vi "Single Measure Reference Query.vi"(8 "error in":errorcluster, 11 "Instrument Handle In":i32) -> (0 "error out":errorcluster, 1 "Low Reference":dbl, 2 "Mid Reference":dbl, 3 "Instrument Handle Out":i32, 5 "High Reference":dbl)   [LabVIEW 8.6, in "ZTScopeM.lvlib"]
doc: "Query the voltage threshold levels for measurements.\nValues may be in either volts or percent depending on the reference method."
uses:
  ZTScopeM.lvlib
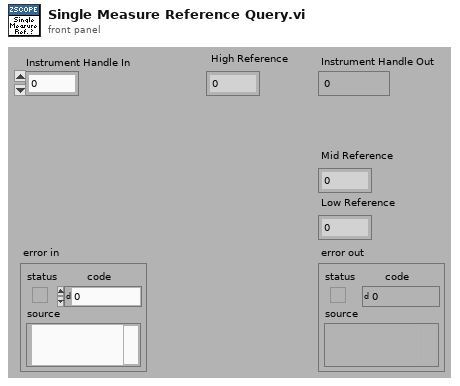
[diagram p1: front panel]
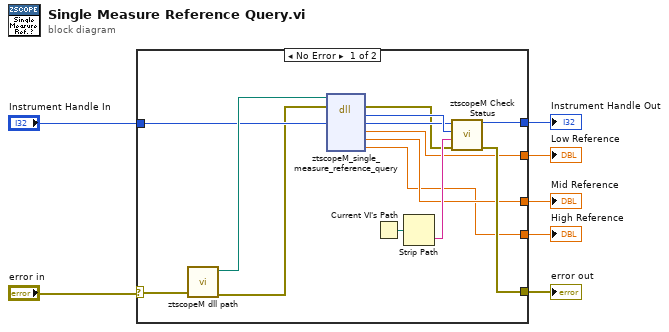
[diagram p0: block diagram]
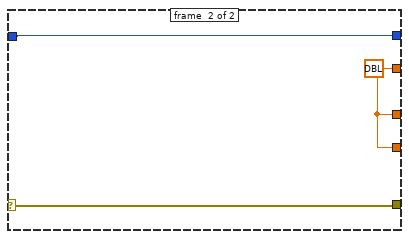
[diagram p2: hidden frame]
diagram:
  n1 = case shown="No Error" "error in" {
    selector: "error in" -> [w12 w24]
    tunnel: [w16 w24] -> w6
    tunnel: [w17 w22] -> w5
    tunnel: [w15 w23] -> w4
    tunnel: [w14 w23] -> w3
    tunnel: [w13 w23] -> w2
    tunnel: "Instrument Handle In" -> [w10 w22]
    frame #0 {
      n2 = call "ztscopeM dll path.vi"("error in (no error)"=w12) -> ("error out"=w9:errorcluster, "<instrument>.dll path"=w11:path)  [unwired: 9 in]
      n3 = dll-call lib="C:/Program Files (x86)/National Instruments/LabVIEW 2013/instr.lib/ztscopem/ztscopeM.dll" fn="ztscopeM_single_measure_reference_query"(path in=w11, error in=w9, "instrumentHandle"=w10) -> (error out=w8:errorcluster, w21:i32, "instrumentHandle"=w20:i32, "lowReference"=w15:dbl, "midReference"=w14:dbl, "highReference"=w13:dbl)  [unwired: 1 in, 4 out]
      n4 = Current VI's Path() -> (path=w19:path)
      n5 = Strip Path(path=w19) -> (name=w18:string)  [unwired: 1 out]
      n6 = call "ztscopeM Check Status.vi"("error in"=w8, "name of VI"=w18, "status (return code)"=w21, "instrument handle in"=w20) -> ("error out"=w16:errorcluster, "instrument handle out"=w17:i32)  [unwired: 2 out]
    }
    frame #1 {
      w23 = dbl ? ("lowReference")
    }
  }
  "Instrument Handle Out" <- w5
  "error out" <- w6
  "Low Reference" <- w4
  "Mid Reference" <- w3
  "High Reference" <- w2
